vi "RT Driver VI.vi"(7 "Operation":T1, 11 "Device Reference in":T2 format="%.0x") -> (0 "Error Code":i32)   [LabVIEW 2019, in "DSF Engine.lvlib"]
uses:
  DSF Engine.lvlib
  VeriStand DSF/VeriStand DSF.lvclass
  <vilib>/NI VeriStand/Custom Device API/Global Data Refs.vi
  <vilib>/NI VeriStand/Custom Device API/Custom Device API.lvlib
  Shared/DSF Shared.lvlib
  DSF Core.lvlibp/Classes/Thread/Thread Options.ctl
  State Data.ctl
  <vilib>/NI VeriStand/Custom Device API/Custom Device Item Ref.ctl
  <vilib>/NI VeriStand/Custom Device API/Hardware Interface Driver VI Operation.ctl
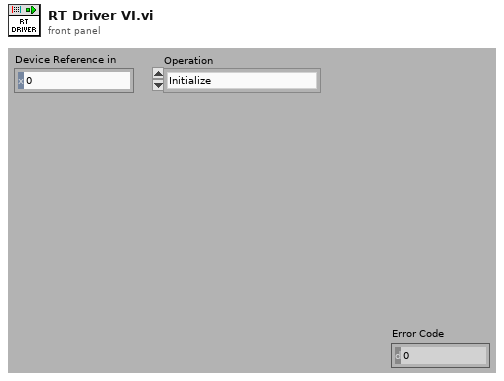
[diagram p1: front panel]
types:
  T1 = typedef "Custom Device API.lvlib/Hardware Interface Driver VI Operation.ctl" = enum16{"Initialize", "Start", "Read Data from HW", "Write Data to HW", "Close"}
  T2 = typedef "Custom Device API.lvlib/Custom Device Item Ref.ctl" = u64
  T3 = typedef "DSF Engine.lvlib/State Data.ctl" = cluster{"show error dialog":bool}
  T4 = typedef "DSF Core.lvlibp/Thread.lvclass/Thread Options.ctl" = cluster{"Show FP On Call":bool, "Close FP After Call":bool, "Allow Debugging":bool}
  T5 = typedef "DSF Core.lvlibp/Framework.lvclass/Framework Options.ctl" = cluster{"FIFO Options":T6, "Thread Options":T4, "Plugin Options":T7, "Performance Options":T8, "Data Server Options":T9}
  T6 = typedef "DSF Core.lvlibp/Framework.lvclass/DSF FIFO Options.ctl" = cluster{"Infinite Timeouts":bool}
  T7 = typedef "DSF Core.lvlibp/Framework.lvclass/DSF Plugin Options.ctl" = cluster{"Default Components":bool}
  T8 = typedef "DSF Core.lvlibp/DSF Performance Options.ctl" = cluster{"Measure Period":bool, "Measure Rx/Tx Duration":bool}
  T9 = typedef "DSF Core.lvlibp/Framework.lvclass/Data Server Options.ctl" = cluster{"Enable Data Server":bool, "Period":u32}
  T10 = typedef "Custom Device API.lvlib/Data Table Ref.ctl" = cluster{"Ptr.Beg":u64, "Ptr.End":u64}
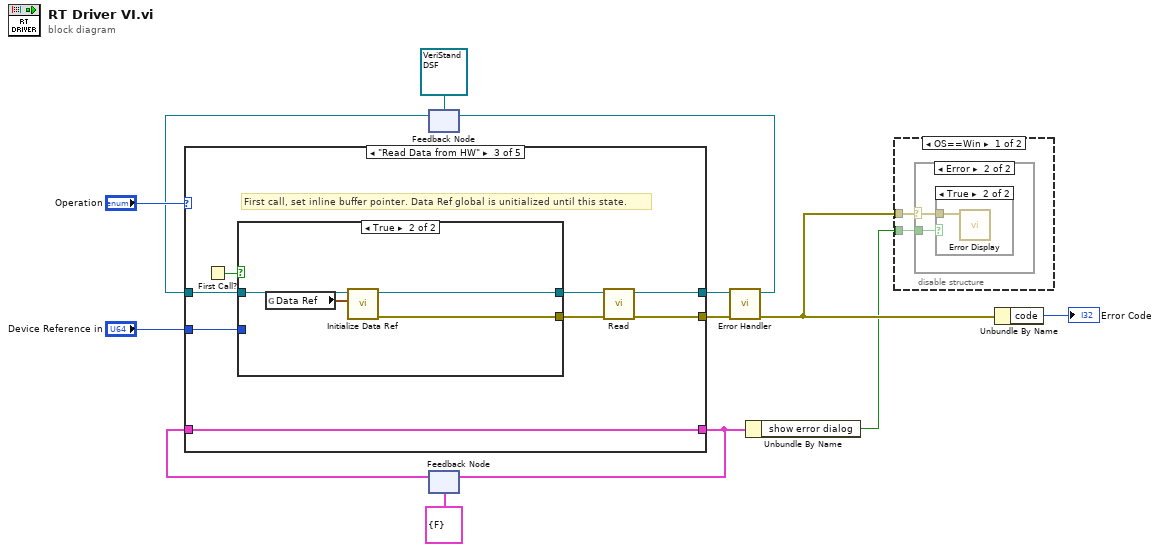
[diagram p0: block diagram]
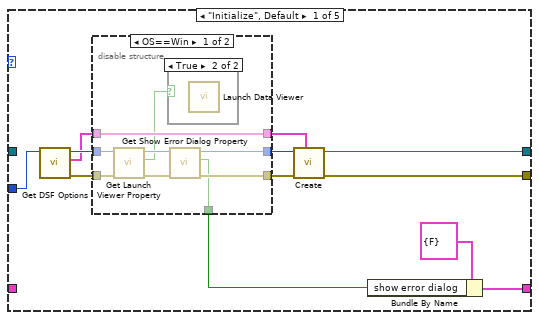
[diagram p2: hidden frame]
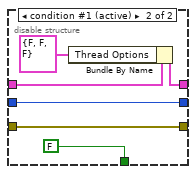
[diagram p4: hidden frame]
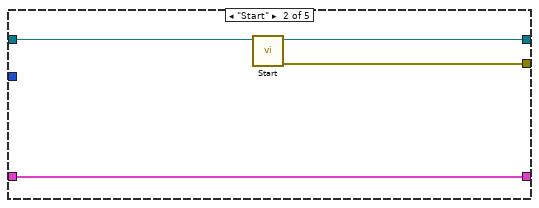
[diagram p5: hidden frame]
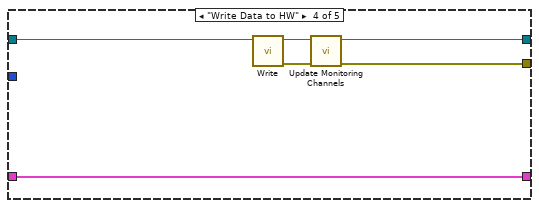
[diagram p7: hidden frame]
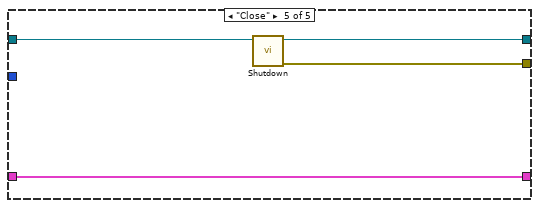
[diagram p8: hidden frame]
diagram:
  n1 = feedback #1(refnum<class "VeriStand DSF.lvclass"> refnum ("Data Sharing Framework Engine.lvlib:VeriStand Data Sharing Framework.lvclass")) -> (w10:refnum<class "VeriStand DSF.lvclass">)
  n2 = feedback #2(T3 {"show error dialog"=FALSE} ("state data")) -> (w8:T3)
  n3 = case shown="\"Read Data from HW\"" "Operation" {
    tunnel: [w25 w43 w50 w59 w65] -> w6
    tunnel: w10 -> [_ w44 w51 w63 w67]
    tunnel: "Device Reference in" -> [w24 _ w46 _ _]
    tunnel: [w14 w42 w47 w58 w66] -> w7
    tunnel: [w21 w41 w45 w62 w64] -> w3
    tunnel: w8 -> [_ w41 w45 w62 w64]
    frame "Initialize", Default {
      n4 = call "Get DSF Options.vi"("Item Ref in"=w24) -> ("error out"=w20:errorcluster, "options"=w15:T5, "Item Ref out"=w19:T2)  [unwired: 8 in]
      n5 = disable-structure shown="OS==Win" {
        disable-tunnel: [w29 w38] -> w23
        disable-tunnel: w15 -> [w29 w39]
        disable-tunnel: w20 -> [w32 w36]
        disable-tunnel: w19 -> [w33 w37]
        disable-tunnel: [w34 w37] -> w18
        disable-tunnel: [w27 w36] -> w17
        disable-tunnel: [w26 FALSE ("launch data viewer")] -> w16
        frame condition #0 {
          n6 = call "Get Launch Viewer Property.vi"("error in (no error)"=w32, "Item Ref in"=w33) -> ("error out"=w30:errorcluster, "launch viewer"=w28:bool, "Item Ref out"=w31:T2)  [unwired: 7 in]
          n7 = case shown="True" w28 {
            frame False {
            }
            frame True {
              n8 = call "Launch Data Viewer.vi"() -> ()  [unwired: 11 in, 1 out]
            }
          }
          n9 = call "Get Show Error Dialog Property.vi"("error in (no error)"=w30, "Item Ref in"=w31) -> ("error out"=w27:errorcluster, "show error dialog"=w26:bool, "Item Ref out"=w34:T2)  [unwired: 7 in]
        }
        frame condition #1 (active) {
          n10 = Bundle By Name(cluster=w39, "Thread Options"=T4 {"Show FP On Call"=FALSE, "Close FP After Call"=FALSE, "Allow Debugging"=FALSE}) -> (w38:T5)
        }
      }
      n11 = call "Create.vi"("options"=w23, "error in (no error)"=w17, "Device Item Ref"=w18) -> ("error out"=w14:errorcluster, "VeriStand Framework"=w25:refnum<class "VeriStand DSF.lvclass">)  [unwired: 7 in]
      n12 = Bundle By Name(cluster=T3 {"show error dialog"=FALSE} ("state data"), "show error dialog"=w16) -> (w21:T3)
    }
    frame "Start" {
      n13 = call-dynamic "Start.vi"("VeriStand Data Sharing Framework in"=w44) -> ("error out"=w42:errorcluster, "VeriStand Data Sharing Framework out"=w43:refnum<class "VeriStand DSF.lvclass">)  [unwired: 9 in]
    }
    frame "Read Data from HW" {
      # "First call, set inline buffer pointer. Data Ref global is unitialized until this state."
      n14 = First Call?() -> (First Call?: T/F=w52:bool)
      n15 = case shown="True" w52 {
        tunnel: w51 -> [w53 w57]
        tunnel: [w53 w55] -> w49
        tunnel: [_ w54] -> w48
        tunnel: w46 -> [_ _]
        frame False {
        }
        frame True {
          n16 = global read "Global Data Refs.vi" "Data Ref"() -> (w56:T10)
          n17 = call "Initialize Data Ref.vi"("Data Ref"=w56, "VeriStand DSF in"=w57) -> ("error out"=w54:errorcluster, "VeriStand DSF out"=w55:refnum<class "VeriStand DSF.lvclass">)  [unwired: 8 in]
        }
      }
      n18 = call "Read.vi"("error in (no error)"=w48, "VeriStand DSF in"=w49) -> ("error out"=w47:errorcluster, "VeriStand DSF out"=w50:refnum<class "VeriStand DSF.lvclass">)  [unwired: 8 in]
    }
    frame "Write Data to HW" {
      n19 = call "Write.vi"("VeriStand DSF in"=w63) -> ("error out"=w60:errorcluster, "VeriStand DSF out"=w61:refnum<class "VeriStand DSF.lvclass">)  [unwired: 9 in]
      n20 = call "Update Monitoring Channels.vi"("error in (no error)"=w60, "VeriStand DSF in"=w61) -> ("error out"=w58:errorcluster, "VeriStand DSF out"=w59:refnum<class "VeriStand DSF.lvclass">)  [unwired: 8 in]
    }
    frame "Close" {
      n21 = call-dynamic "Shutdown.vi"("VeriStand Data Sharing Framework in"=w67) -> ("error out"=w66:errorcluster, "VeriStand Data Sharing Framework out"=w65:refnum<class "VeriStand DSF.lvclass">)  [unwired: 9 in]
    }
  }
  n22 = feedback-in #2(w3) -> ()
  n23 = call "Error Handler.vi"("error in (no error)"=w7, "Framework in"=w6) -> ("error out"=w5:errorcluster, "Framework out"=w1:refnum<class "VeriStand DSF.lvclass">)  [unwired: 8 in]
  n24 = feedback-in #1(w1) -> ()
  n25 = Unbundle By Name(w3) -> ("show error dialog"=w2:bool)
  n26 = disable-structure shown="OS==Win" {
    disable-tunnel: w5 -> [w69 _]
    disable-tunnel: w2 -> [w68 _]
    frame condition #0 {
      n27 = case shown="Error" w69 {
        selector: w69 -> [_ w71]
        tunnel: w68 -> [_ w70]
        frame No Error {
        }
        frame Error {
          n28 = case shown="True" w70 {
            tunnel: w71 -> [_ w72]
            frame False {
            }
            frame True {
              n29 = call "Error Display.vi"("error"=w72) -> ()  [unwired: 11 in]
            }
          }
        }
      }
    }
    frame condition #1 (active) {
    }
  }
  n30 = Unbundle By Name(w5) -> ("code"=→"Error Code":i32)
